vi "Configure Channel Settings.vi"(0 "VISA resource name":refnum<visa-resource-name>, 1 "Base Line Offset (V)":dbl, 3 "Selection Scale":u8(ring) items=["Value", "Minimum", "Maximum", "Default"], 5 "Amplitude Scale (%)":dbl=100.0, 6 "Selection Skew":u8(ring) items=["Value", "Minimum", "Maximum", "Default"], 7 "Channel (0: Channel 1)":u16(ring) items=["Channel 1", "Channel 2", "Channel 3", "Channel 4", "Channel 5", "Channel 6", "Channel 7", "Channel 8"], 9 "Skew (s)":dbl, 10 "Selection Base Line Offset(V)":u8(ring) items=["Value", "Minimum", "Maximum", "Default"], 11 "error in (no error)":errorcluster, 12 "Output Impedance":u8(ring) items=["50 Ohm", "Low"], 14 "Polarity":u8(ring) items=["Positive", "Negative"]) -> (4 "VISA resource name out":refnum<visa-resource-name>, 15 "error out":errorcluster)   [LabVIEW 2020, in "Active Technologies AWG3000.lvlib"]
uses:
  Active Technologies AWG3000.lvlib
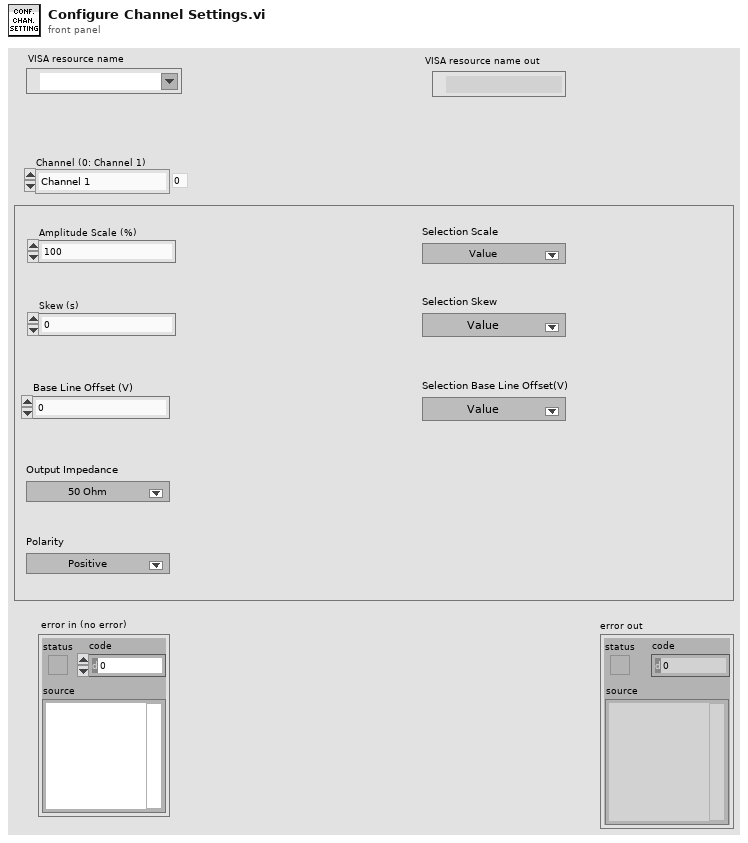
[diagram p1: front panel]
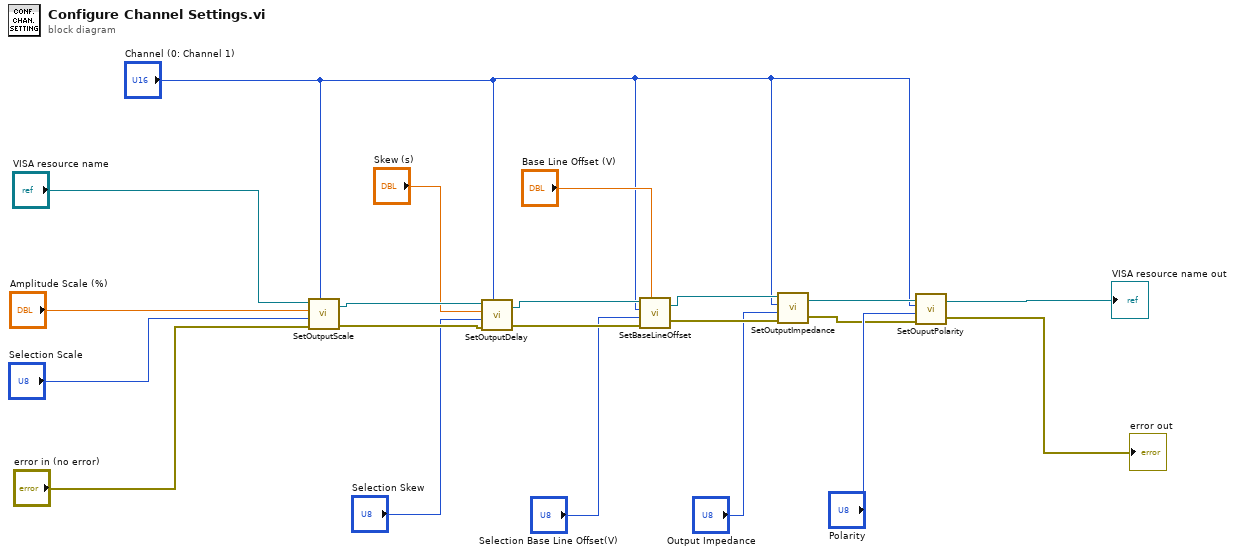
[diagram p0: block diagram]
diagram:
  n1 = call "SetOutputScale.vi"("VISA resource name"="VISA resource name", "Amplitude Scale (%)"="Amplitude Scale (%)", "Selection"="Selection Scale", "error in (no error)"="error in (no error)", "Channel (0: Channel 1)"="Channel (0: Channel 1)") -> ("VISA resource name out"=w17:refnum<visa-resource-name>, "error out"=w15:errorcluster)
  n2 = call "SetOutputDelay.vi"("VISA resource name"=w17, "Skew (s)"="Skew (s)", "Selection"="Selection Skew", "error in (no error)"=w15, "Channel (0: Channel 1)"="Channel (0: Channel 1)") -> ("VISA resource name out"=w13:refnum<visa-resource-name>, "error out"=w12:errorcluster)
  n3 = call "SetBaseLineOffset.vi"("VISA resource name"=w13, "Channel (0: Channel 1)"="Channel (0: Channel 1)", "Selection"="Selection Base Line Offset(V)", "error in (no error)"=w12, "Base Line Offset (V)"="Base Line Offset (V)") -> ("VISA resource name out"=w9:refnum<visa-resource-name>, "error out"=w8:errorcluster)
  n4 = call "SetOutputImpedance.vi"("error in (no error)"=w8, "Output Impedance"="Output Impedance", "Channel (0: Channel 1)"="Channel (0: Channel 1)", "VISA resource name"=w9) -> ("error out"=w3:errorcluster, "VISA resource name out"=w6:refnum<visa-resource-name>)
  n5 = call "SetOuputPolarity.vi"("error in (no error)"=w3, "Polarity"="Polarity", "Channel (0: Channel 1)"="Channel (0: Channel 1)", "VISA resource name"=w6) -> ("error out"=→"error out":errorcluster, "VISA resource name out"=→"VISA resource name out":refnum<visa-resource-name>)
